vi "Normalized Axes Logic.vi"(8 "axis":dbl[](array[numeric]), 11 "axis in":i32) -> (3 "axis out":dbl)   [LabVIEW 2012]
doc: "This VI contains specific logic to update an individual axis' minimum and maximum range.\nNote that the polarity of 'axis in' is used to determine the exact element within 'axis' to serve as the divisor within the normalization process.\nRuffin"
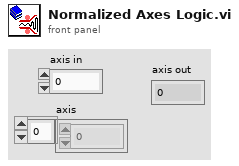
[diagram p1: front panel]
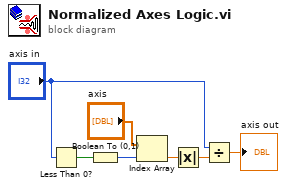
[diagram p0: block diagram]
diagram:
  n1 = Less Than 0?(x="axis in") -> (x < 0?=w6:bool)
  n2 = Boolean To (0,1)(Boolean=w6) -> (0, 1=w7:i16)
  n3 = Index Array(array="axis", index=w7) -> (element=w5:dbl)
  n4 = Absolute Value(x=w5) -> (abs(x)=w4:dbl)
  n5 = Divide(x="axis in", y=w4) -> (x/y=→"axis out":dbl)
